vi "ACT_Loop_Single Test.vi"() -> ()   [LabVIEW 2023]
uses:
  Cluster_CMD_ACT_Data.ctl
  Shared Code/TypeDefs/ENUM_CMD_Mode Select.ctl
  Shared Code/TypeDefs/Cluster_CMD_Direction Data.ctl
  Shared Code/TypeDefs/Cluster_Module Velocity-Direction-Rotations.ctl
  Shared Code/TypeDefs/Level_Velocity plus-minus 1.ctl
  Shared Code/TypeDefs/Dial_Compase heading unit circle CCW positive.ctl
  Shared Code/TypeDefs/Cluster_X-Y.ctl
  <vilib>/Rock Robotics/WPI/ThirdParty/REV Robotics/REVLib/Typedef/Spark MAX Control Type.ctl
  Type Defs/ENUM_Steer Mode Select.ctl
  Shared Code/TypeDefs/Cluster_Swerve 4 Steer and Velocity.ctl
  Shared Code/TypeDefs/Cluster_Swerve Actual Settings.ctl
  Shared Code/TypeDefs/Cluster_Module Actual Settings.ctl
  Shared Code/TypeDefs/Dial_Actual Direction.ctl
  ENUM_ACT_State.ctl
  <vilib>/Rock Robotics/WPI/MotorControl/WPI_MotorControlDeviceRef.ctl
  <vilib>/Rock Robotics/WPI/MotorControl/WPI_MotorControlType.ctl
  <vilib>/Rock Robotics/SystemInterfaces/DIO/FPGA_DIOPWMChannel.ctl
  <vilib>/Rock Robotics/WPI/PWM/WPI_PWMDeadband.ctl
  <vilib>/Rock Robotics/SystemInterfaces/DIO/FPGA_DIOChannel.ctl
  Shared Code/TypeDefs/ENUM_Module Position.ctl
  Type Defs/Cluster_Avoid Zone.ctl
  Shared Code/TypeDefs/Cluster_Config_Swerve Drive Parameters.ctl
  Type Defs/Cluster_Length and Width.ctl
  Shared Code/TypeDefs/Cluster_Config_SwerveParam Steer.ctl
  Shared Code/TypeDefs/Cluster_Config_SwerveParam Drive.ctl
  <vilib>/Rock Robotics/WPI/ThirdParty/Phoenix-LabVIEW/CANCoder/Controls/CTRE_Phoenix_CANcoder_DeviceRef.ctl
  ENUM_ACT_Action.ctl
  RoboRIO Utilities/Global_STOP.vi
  Global_CMD_ACT_Data In.vi
  PigeonIMU/Global_SEN_Data Out.vi
  <vilib>/Rock Robotics/WPI/ThirdParty/Phoenix-LabVIEW/CANCoder/Get/CTRE_Phoenix_CANcoder_GetSensorData.vi
  Global_ACT_Data Out.vi
  SwerveDrive_ACT_ts.lvlib
  PigeonIMU/PigeonIMU_SEN_ts.lvlib
panel:
  in  "OVERIDE Tab":enum32{"Teleop-Auto", "Move", "Stop"}(tab)
  in  "SEND CMD(Momentry)":bool
  in  "Rotation Reduction 1-0":dbl=0.5
  in  "Orientation Robot(t) Field(f)":bool=TRUE
  in  "Direction":T1 {"Rotate(Yaw) CCW 1 CW -1" scale=1.0..-1.0; "Traverse"."Angle" scale format="%.3f"; "Traverse"."Velocity" scale=-1.0..1.0 scale format="%.1f"}
  in  "Max Translation Speed (ft/sec)":dbl
  out "Cancoder Values":dbl[](array[numeric]) format="%#.6f"
  out "Steer values":dbl[](array[numeric]) format="%.6g"
  out "unit circ Steer values":dbl[](array[numeric]) format="%.6g"
  out "unit circ Cancoder values":dbl[](array[numeric]) format="%#.6f"
  out "Yaw":T4 scale format="%.3f"
  out "Swerve SET Actual":T5 {"Back Right"."Encoder" format="%.2f"; "Back Right"."Direction" scale format="%.3f"; "Back Right"."Velocity" format="%.2f"; "Back Left"."Encoder" format="%.2f"; "Back Left"."Direction" scale format="%.3f"; "Back Left"."Velocity" format="%.2f"; "Front Left"."Encoder" format="%.2f"; "Front Left"."Direction" scale format="%.3f"; "Front Left"."Velocity" format="%.2f"; "Front Right"."Encoder" format="%.2f"; "Front Right"."Direction" scale format="%.3f"; "Front Right"."Velocity" format="%.2f"}
  out "calc time":dbl
  out "Swerve Set":T8 {"Back Right"."Angle" scale format="%.3f"; "Back Right"."Velocity" scale=-1.0..1.0 scale format="%.1f"; "Back Left"."Angle" scale format="%.3f"; "Back Left"."Velocity" scale=-1.0..1.0 scale format="%.1f"; "Front Left"."Angle" scale format="%.3f"; "Front Left"."Velocity" scale=-1.0..1.0 scale format="%.1f"; "Front Right"."Angle" scale format="%.3f"; "Front Right"."Velocity" scale=-1.0..1.0 scale format="%.1f"}
  out "Max Velocity(RPM)":dbl=200.0
  out "Steer Mode":T9
  out "Max Velocity FPS":dbl=2.0
  out "Drive Control Mode":T10
  out "Input CMD":T11 {"Auto Angle" scale format="%.3f"; "Direction"."Rotate(Yaw) CCW 1 CW -1" scale=1.0..-1.0; "Direction"."Traverse"."Angle" scale format="%.3f"; "Direction"."Traverse"."Velocity" scale=-1.0..1.0 scale format="%.1f"}
  out "Cycle Time (S)":dbl format="%.3g"
  # "TeleOp or Auto Control"
  # "STOP"
  # "\"Front\" of Robot"
  # "X"
  # "+CCW"
  # "Y"
  # "(0,0)"
  # "\"Front\" of Robot"
  # "Right Hand Rule"
  # "X"
  # "+CCW"
  # "Y"
  # "(0,0)"
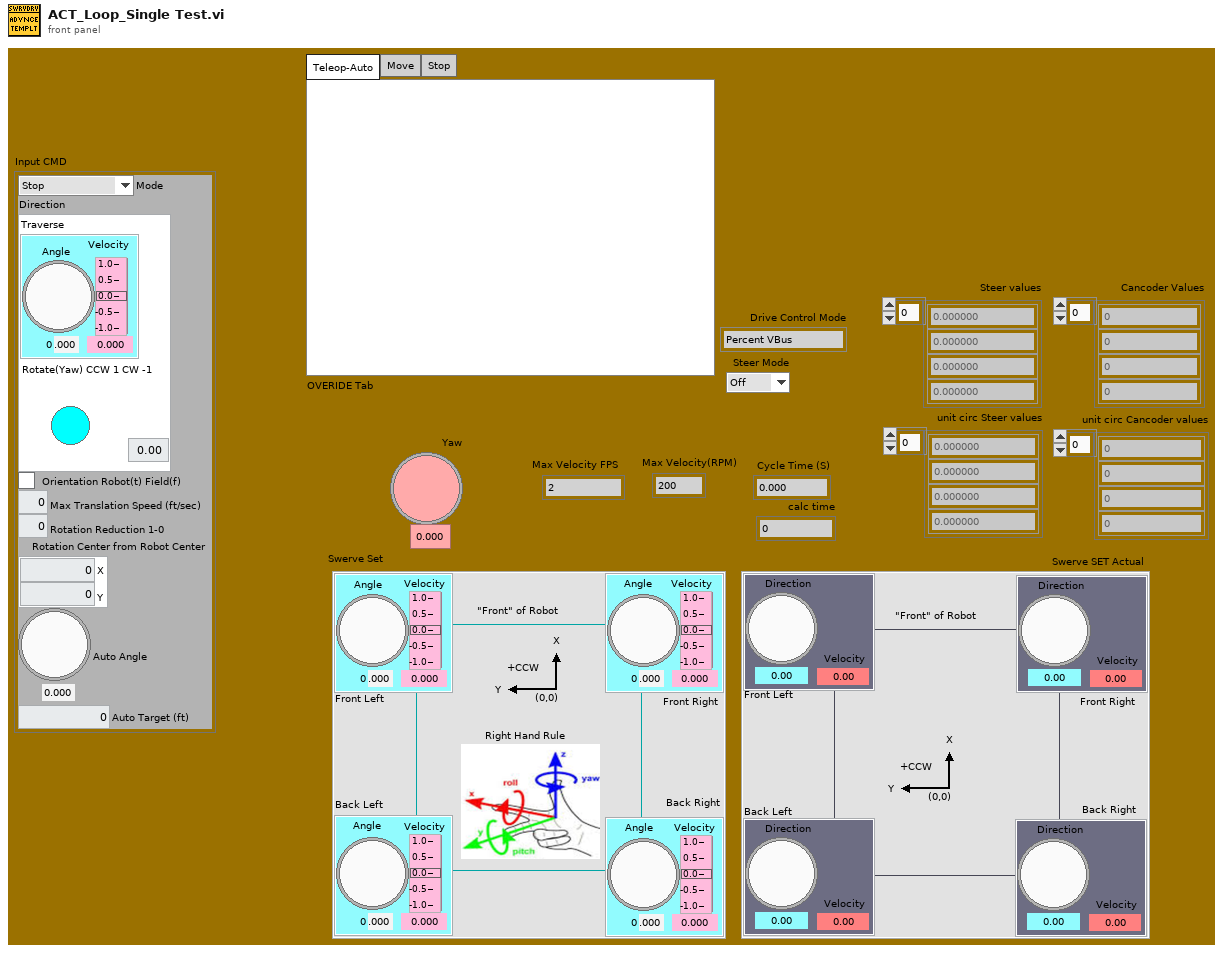
[diagram p1: front panel]
types:
  T1 = typedef "Cluster_CMD_Direction Data.ctl" = cluster{"Traverse":T2, "Rotate(Yaw) CCW 1 CW -1":dbl}
  T2 = typedef "Cluster_Module Velocity-Direction-Rotations.ctl" = cluster{"Velocity":T3, "Angle":T4, "Rotations Count":dbl}
  T3 = typedef "Level_Velocity plus-minus 1.ctl" = dbl
  T4 = typedef "Dial_Compase heading unit circle CCW positive.ctl" = dbl
  T5 = typedef "Cluster_Swerve Actual Settings.ctl" = cluster{"Front Right":T6, "Front Left":T6, "Back Left":T6, "Back Right":T6}
  T6 = typedef "Cluster_Module Actual Settings.ctl" = cluster{"Velocity":dbl, "Direction":T7, "Encoder":dbl}
  T7 = typedef "Dial_Actual Direction.ctl" = dbl
  T8 = typedef "Cluster_Swerve 4 Steer and Velocity.ctl" = cluster{"Front Right":T2, "Front Left":T2, "Back Left":T2, "Back Right":T2}
  T9 = typedef "ENUM_Steer Mode Select.ctl" = enum16{"Off", "Hold", "Steer"}
  T10 = typedef "Spark MAX Control Type.ctl" = enum16{"Percent VBus", "Voltage", "Velocity", "Position", "Smart Motion", "Current", "Smart Velocity"}
  T11 = typedef "SwerveDrive_ACT_ts.lvlib/Cluster_CMD_ACT_Data.ctl" = cluster{"Mode":T12, "Direction":T1, "Orientation Robot(t) Field(f)":bool, "Max Translation Speed (ft/sec)":dbl, "Rotation Reduction 1-0":dbl, "Rotation Center from Robot Center":T13, "Auto Angle":T4, "Auto Target (ft)":dbl}
  T12 = typedef "ENUM_CMD_Mode Select.ctl" = enum16{"Stop", "Move", "Turret Manual"}
  T13 = typedef "Cluster_X-Y.ctl" = cluster{"X":dbl, "Y":dbl}
  T14 = typedef "CTRE_Phoenix_CANcoder_DeviceRef.ctl" = cluster{"DeviceStatus":errorcluster, "Device Number":u8, "Handle":u64, "UsageFrame":u32, "Library Path":path}
  T15 = typedef "Cluster_Config_Swerve Drive Parameters.ctl" = cluster{"SwerveParam Ver":u64, "Frame":T16, "Steer":T17, "Drive":T18}
  T16 = typedef "Cluster_Length and Width.ctl" = cluster{"Length":dbl, "Width":dbl}
  T17 = typedef "Cluster_Config_SwerveParam Steer.ctl" = cluster{"CPR":dbl}
  T18 = typedef "Cluster_Config_SwerveParam Drive.ctl" = cluster{"CPR":dbl, "RevMotor/Wheel":dbl, "Wheel Diameter (in)":dbl}
  T19 = typedef "Cluster_Avoid Zone.ctl" = cluster{"pos 1":dbl, "pos 2":dbl}
  T20 = typedef "ENUM_Module Position.ctl" = enum16{"Left-Front", "Right-Front", "Left-Back", "Right-Back"}
  T21 = typedef "WPI_MotorControlDeviceRef.ctl" = cluster{"DeviceStatus":errorcluster, "Type":T22, "PWM":cluster{"PWM Channel":T23, "DeadBand":T24}, "CAN":cluster{"Device Number":u8, "SetOutput VI Ref":variant, "GetOutput VI Ref":variant, "Enable VI Ref":variant, "Disable VI Ref":variant, "Data":variant}, "Invert":bool, "DIO PWM":cluster{"PWM \"Enable\" Channel":T23, "DIOChannel":T25, "PWM Rate":dbl}}
  T22 = typedef "WPI_MotorControlType.ctl" = enum16{"PWM", "CAN", "DIO PWM"}
  T23 = typedef "FPGA_DIOPWMChannel.ctl" = enum8{"PWM 0", "PWM 1", "PWM 2", "PWM 3", "PWM 4", "PWM 5", "PWM 6", "PWM 7", "PWM 8", "PWM 9", "PWM MXP 0", "PWM MXP 1", "PWM MXP 2", "PWM MXP 3", "PWM MXP 4", "PWM MXP 5", "PWM MXP 6", "PWM MXP 7", "PWM MXP 8", "PWM MXP 9", "Invalid"}
  T24 = typedef "WPI_PWMDeadband.ctl" = cluster{"Name":string, "maxPositivePwm":i32, "minPositivePwm":i32, "centerPwm":i32, "maxNegativePwm":i32, "minNegativePwm":i32, "angularRange":u16}
  T25 = typedef "FPGA_DIOChannel.ctl" = enum8{"DIO 0", "DIO 1", "DIO 2", "DIO 3", "DIO 4", "DIO 5", "DIO 6", "DIO 7", "DIO 8", "DIO 9", "DIO MXP 0", "DIO MXP 1", "DIO MXP 2", "DIO MXP 3", "DIO MXP 4", "DIO MXP 5", "DIO MXP 6", "DIO MXP 7", "DIO MXP 8", "DIO MXP 9", "DIO MXP 10", "DIO MXP 11", "DIO MXP 12", "DIO MXP 13", "DIO MXP 14", "DIO MXP 15", "SPI Port CS1", "SPI Port CS2", "SPI Port CS3", "SPI Port MISO", "SPI Port MOSI", "Invalid"}
  T26 = typedef "SwerveDrive_ACT_ts.lvlib/ENUM_ACT_State.ctl" = enum16{"Startup", "Stopping", "Moving", "Shutdown"}
  T27 = typedef "SwerveDrive_ACT_ts.lvlib/ENUM_ACT_Action.ctl" = enum16{"No Action", "Reset Time", "Reset All", "2 Pos Set Direction", "2 Pos Set Speed", "Record Data", "Set Move from Values", "Reset Steer to Absolute"}
  T28 = cluster{"Motor List":T20[], "Drive Refs":T21[], "Steer Refs":T21[], "State":T26, "Previous State":T26, "Current Time":timestamp, "Previous Time":timestamp, "Start Time":timestamp, "Target Time (ms)":u32, "Cycle Time(S)":dbl, "ACT Input":T11, "Drive Control Mode":T10, "Drive PID Slot":i32, "Steer Position Values":dbl[], "Drive Velocity Values":dbl[], "Steer Position Times":dbl[], "Drive Velocity Times":dbl[], "Stream":bool, "Drive Output Times":dbl[], "Drive Output Values":dbl[], "Zero Start Steer Positions":dbl[], "Steer Mode":T9, "Max Velocity RPM":dbl, "Avoid Zone":T19, "Swerve Set":T8, "calc Start Time":dbl, "Compass Heading":T4, "Swerve Config ":T15, "Team Folder":path, "Steer Output Times":dbl[], "Can Coder Refs":T14[], "Can Coder Output postions":dbl[]}
  T29 = typedef "Cluster_Unity Yaw-Pitch-Roll.ctl" = cluster{"Yaw":T4, "Pitch":T4, "Roll":T4}
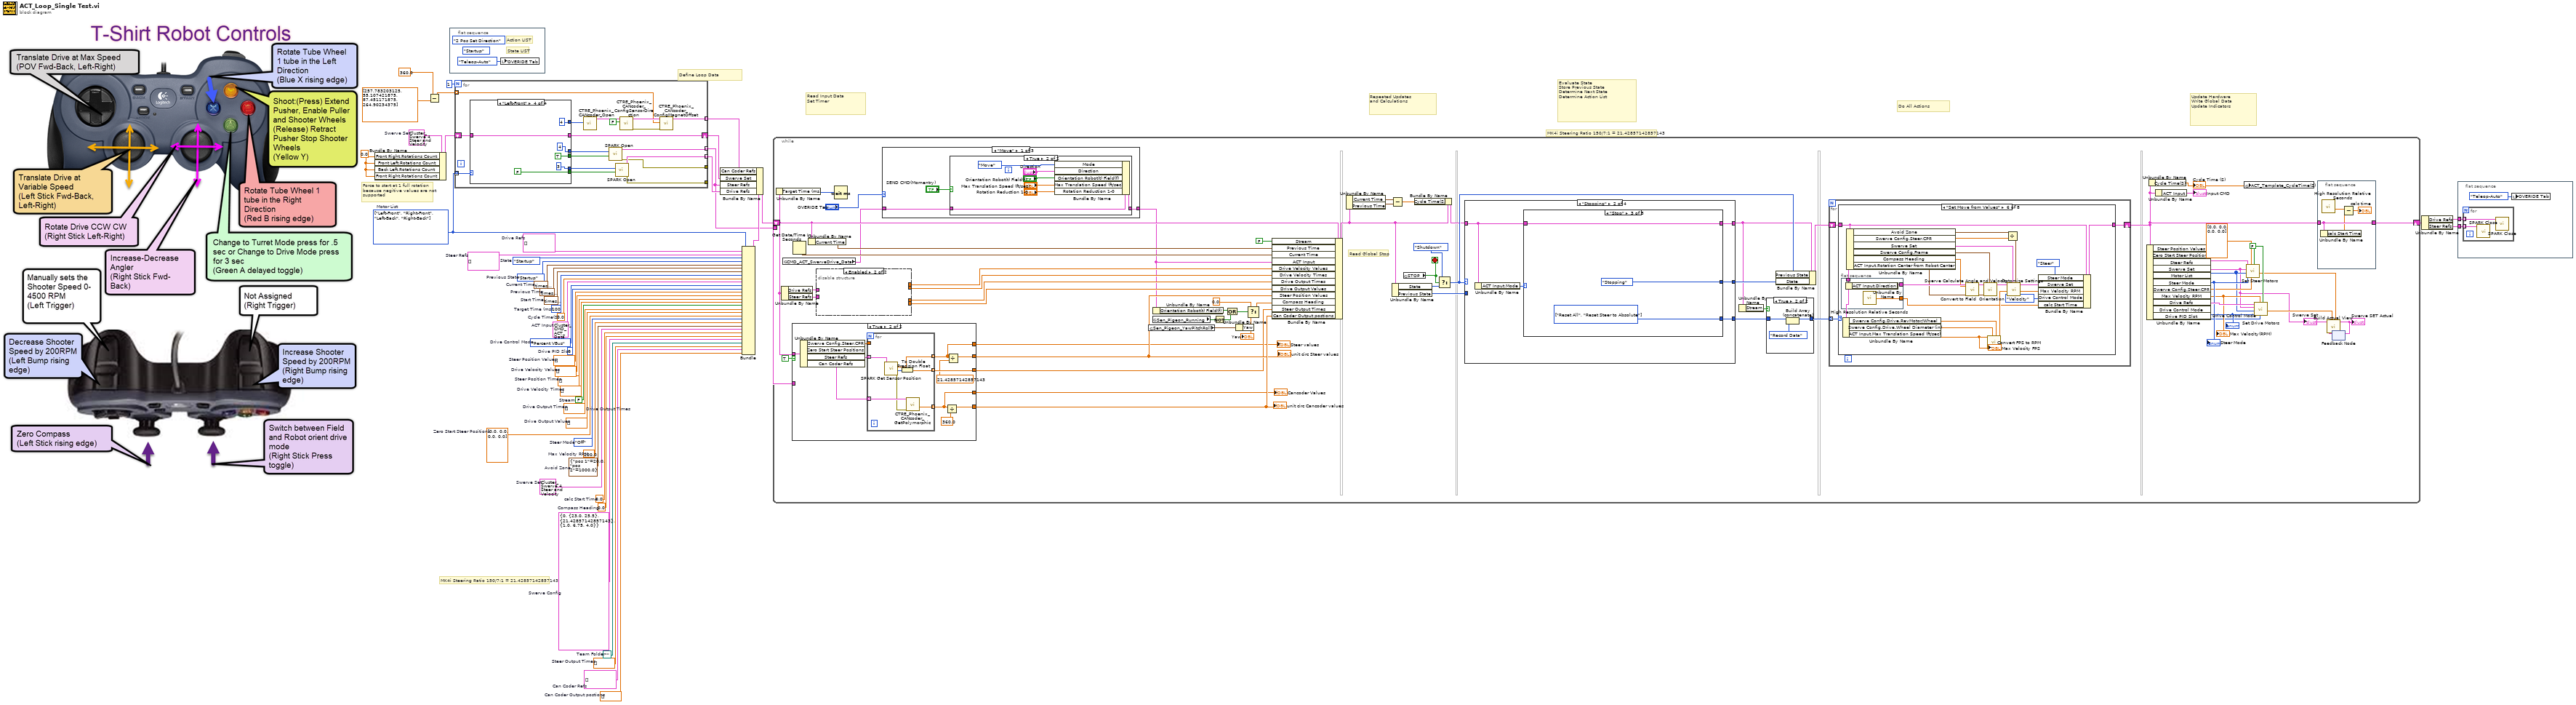
[diagram p0: block diagram]
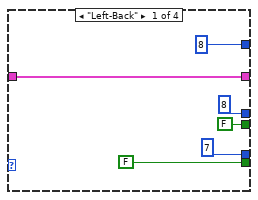
[diagram p2: hidden frame]
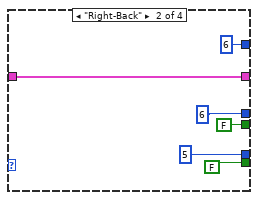
[diagram p3: hidden frame]
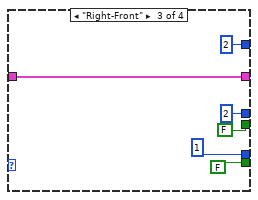
[diagram p4: hidden frame]
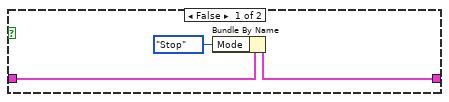
[diagram p5: hidden frame]
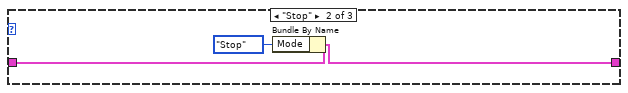
[diagram p6: hidden frame]
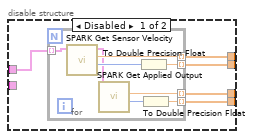
[diagram p8: hidden frame]
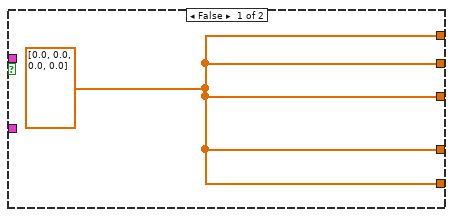
[diagram p9: hidden frame]
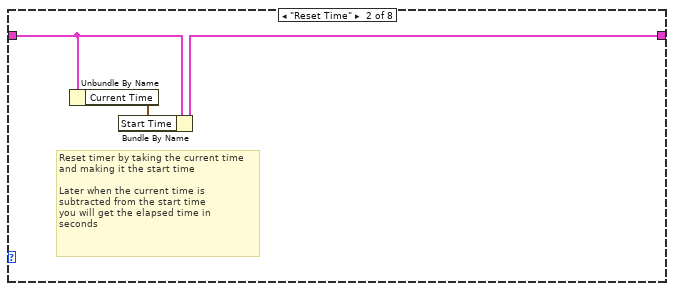
[diagram p12: hidden frame]
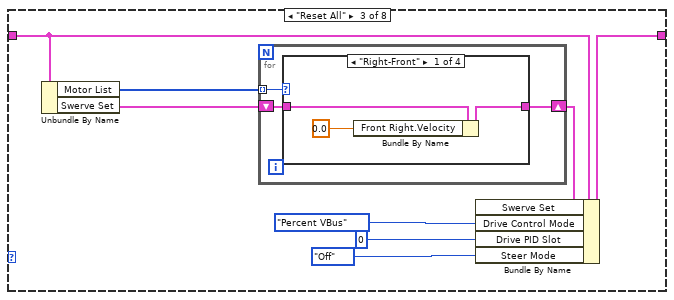
[diagram p13: hidden frame]
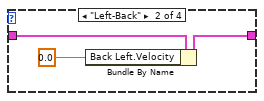
[diagram p14: hidden frame]
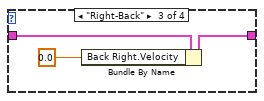
[diagram p15: hidden frame]
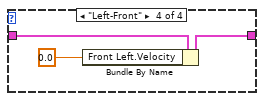
[diagram p16: hidden frame]
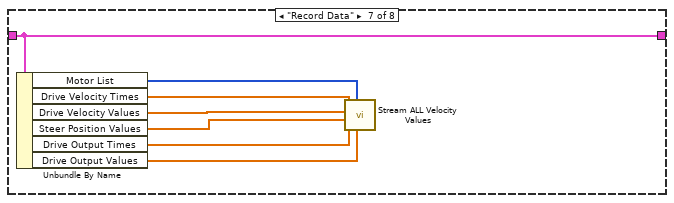
[diagram p19: hidden frame]
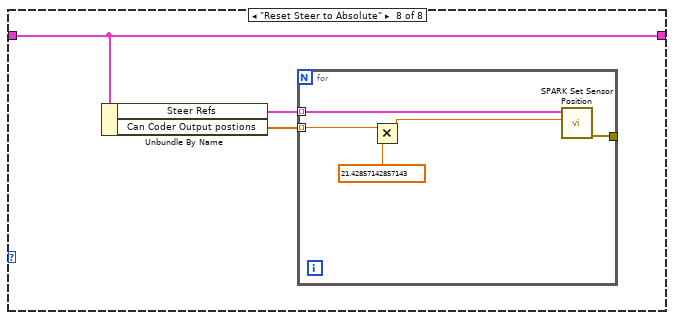
[diagram p20: hidden frame]
diagram:
  w2 = 0.0
  w9 = dbl[] []  # Can Coder Output postions
  w11 = T14[] []  # Can Coder Refs
  w12 = dbl[] []  # Steer Output Times
  (unwired) dbl[] []  # Drive Output Times
  w13 = path ""  # Team Folder
  w14 = T15 {"SwerveParam Ver"=0, "Frame"={"Length"=23.0, "Width"=25.5}, "Steer"={"CPR"=21.42857142857143}, "Drive"={"CPR"=1.0, "RevMotor/Wheel"=6.75, "Wheel Diameter (in)"=4.0}}  # Swerve Config
  w15 = T4 0.0  # Compass Heading
  w16 = 0.0  # calc Start Time
  w4 = T8 {"Front Right"={"Velocity"=0.0, "Angle"=0.0, "Rotations Count"=0.0}, "Front Left"={"Velocity"=0.0, "Angle"=0.0, "Rotations Count"=0.0}, "Back Left"={"Velocity"=0.0, "Angle"=0.0, "Rotations Count"=0.0}, "Back Right"={"Velocity"=0.0, "Angle"=0.0, "Rotations Count"=0.0}}  # Swerve Set
  w18 = T8 {"Front Right"={"Velocity"=0.0, "Angle"=0.0, "Rotations Count"=0.0}, "Front Left"={"Velocity"=0.0, "Angle"=0.0, "Rotations Count"=0.0}, "Back Left"={"Velocity"=0.0, "Angle"=0.0, "Rotations Count"=0.0}, "Back Right"={"Velocity"=0.0, "Angle"=0.0, "Rotations Count"=0.0}}  # Swerve Set
  w19 = T19 {"pos 1"=20.0, "pos 2"=1000.0}  # Avoid Zone
  w20 = T20[] [enum."Left-Front", enum."Right-Front", enum."Left-Back", enum."Right-Back"] items=["Left-Front", "Right-Front", "Left-Back", "Right-Back"]  # Motor List
  w21 = 200.0  # Max Velocity RPM
  w22 = ENUM_Steer_Mode_Select."Off"  # Steer Mode
  w23 = dbl[] [0.0, 0.0, 0.0, 0.0]  # Zero Start Steer Positions
  w24 = dbl[] []  # Drive Output Values
  w25 = dbl[] []  # Drive Output Times
  w26 = FALSE  # Stream
  w27 = dbl[] []  # Drive Velocity Times
  w28 = dbl[] []  # Steer Position Times
  w29 = dbl[] []  # Drive Velocity Values
  w30 = dbl[] []  # Steer Position Values
  w33 = 0  # Drive PID Slot
  w34 = Spark_MAX_Control_Type."Percent VBus"  # Drive Control Mode
  w38 = T21[] []  # Drive Refs
  w39 = T21[] []  # Steer Refs
  w41 = 0.0  # Cycle Time(S)
  w42 = ENUM_ACT_State."Startup"  # Previous State
  w43 = timestamp(0 s since 1904-01-01)  # Previous Time
  w44 = u32 100  # Target Time (ms)
  w45 = T11 {"Mode"=enum."Stop", "Direction"={"Traverse"={"Velocity"=0.0, "Angle"=0.0, "Rotations Count"=0.0}, "Rotate(Yaw) CCW 1 CW -1"=0.0}, "Orientation Robot(t) Field(f)"=FALSE, "Max Translation Speed (ft/sec)"=0.0, "Rotation Reduction 1-0"=0.0, "Rotation Center from Robot Center"={"X"=0.0, "Y"=0.0}, "Auto Angle"=0.0, "Auto Target (ft)"=0.0}  # ACT Input
  w46 = timestamp(0 s since 1904-01-01)  # Start Time
  w47 = timestamp(0 s since 1904-01-01)  # Current Time
  w48 = ENUM_ACT_State."Startup"  # State
  # "Force to start at 1 full rotation\nbecause negitive values are not\nsupported"
  # "MK4i Steering Ratio 150/7:1 = 21.42857142857143"
  # "MK4i Steering Ratio 150/7:1 = 21.42857142857143"
  # "Define Loop Data"
  # "Repeated Updates\nand Calculations"
  # "Read Input Data\nSet Timer"
  # "Evaluate State\nStore Previous State\nDetermine Next State\nDetermine Action List"
  # "Do All Actions"
  # "Update Hardware\nWrite Global Data\nUpdate Indicators"
  n1 = Bundle By Name(cluster=w4, "Front Right.Rotations Count"=w2, "Front Left.Rotations Count"=w2, "Back Left.Rotations Count"=w2, "Front Right.Rotations Count"=w2) -> (w3:T8)
  n2 = Subtract(x=360.0, y=dbl[] [257.783203125, 55.107421875, 87.451171875, 264.90234375] ("Cancoder Values")) -> (x-y=w5:dbl[])
  n3 = flat-sequence {
    frame #0 {
      (unwired) ENUM_ACT_State."Startup" ("State")
      (unwired) ENUM_ACT_Action."2 Pos Set Direction" ("Action")
      # "State LIST"
      # "Action LIST"
      n4 = local write "OVERIDE Tab"(enum32{"Teleop-Auto", "Move", "Stop"}."Teleop-Auto" ("OVERIDE Tab")) -> ()
    }
  }
  n5 = for {
    N: 1 ("Numeric") -> [_]
    tunnel: w20 -> [w67] mode=indexing
    tunnel: [w61] -> w8 mode=indexing
    tunnel: [w64] -> w35 mode=indexing
    shift-right: [w65] -> w17
    shift-left: w3 -> [w66]
    tunnel: [w63] -> _
    tunnel: [w52] -> w10 mode=indexing
    tunnel: [w56] -> _
    tunnel: w5 -> [w50] mode=indexing
    n6 = case shown="\"Left-Front\"" w67 {
      tunnel: [FALSE ("Invert") FALSE ("Invert") FALSE ("Invert") FALSE ("Invert")] -> w62
      tunnel: [u8 7 ("unsigned 8bit integer") u8 5 ("unsigned 8bit integer") u8 1 ("unsigned 8bit integer") u8 3 ("unsigned 8bit integer")] -> w60
      tunnel: w66 -> [w68 w74 w80 w86]
      tunnel: [w68 w74 w80 w86] -> w65
      tunnel: [u8 8 ("Device Number") u8 6 ("Device Number") u8 2 ("Device Number") u8 4 ("Device Number")] -> w59
      tunnel: [FALSE ("Invert") FALSE ("Invert") FALSE ("Invert") TRUE ("Invert")] -> w58
      tunnel: [u8 8 ("Device Number") u8 6 ("Device Number") u8 2 ("Device Number") u8 4 ("Device Number")] -> w57
      frame "Left-Back" {
      }
      frame "Right-Back" {
      }
      frame "Right-Front" {
      }
      frame "Left-Front" {
      }
    }
    n7 = call <vilib>:"CTRE_Phoenix_CANcoder_Open.vi"("Device Number"=w57) -> ("CTRE_CANcoder_DeviceRef"=w55:T14)  [unwired: 9 in, 1 out]
    n8 = call <vilib>:"SPARK Open.vi"("Invert"=w58, "Device Number"=w59) -> ("error out"=w56:errorcluster, "MotorControlDeviceRef"=w61:T21)  [unwired: 8 in]
    n9 = call <vilib>:"SPARK Open.vi"("Invert"=w62, "Device Number"=w60) -> ("error out"=w63:errorcluster, "MotorControlDeviceRef"=w64:T21)  [unwired: 8 in]
    n10 = call <vilib>:"CTRE_Phoenix_CANcoder_ConfigSensorDirection.vi"("Sensor Direction"=FALSE, "CTRE_CANcoder_DeviceRef"=w55) -> ("error out"=w51:errorcluster, "CTRE_CANcoder_DeviceRef"=w53:T14)  [unwired: 8 in]
    n11 = call <vilib>:"CTRE_Phoenix_CANcoder_ConfigMagnetOffset.vi"("error in"=w51, "Magnet Offset (Degrees)"=w50, "CTRE_CANcoder_DeviceRef"=w53) -> ("CTRE_CANcoder_DeviceRef"=w52:T14)  [unwired: 7 in, 1 out]
  }
  n12 = Bundle("Motor List"=w20, "Drive Refs"=w38, "Steer Refs"=w39, "State"=w48, "Previous State"=w42, "Current Time"=w47, "Previous Time"=w43, "Start Time"=w46, "Target Time (ms)"=w44, "Cycle Time(S)"=w41, "ACT Input"=w45, "Drive Control Mode"=w34, "Drive PID Slot"=w33, "Steer Position Values"=w30, "Drive Velocity Values"=w29, "Steer Position Times"=w28, "Drive Velocity Times"=w27, "Stream"=w26, "Drive Output Times"=w25, "Drive Output Values"=w24, "Zero Start Steer Positions"=w23, "Steer Mode"=w22, "Max Velocity RPM"=w21, "Avoid Zone"=w19, "Swerve Set"=w18, "calc Start Time"=w16, "Compass Heading"=w15, "Swerve Config"=w14, "Team Folder"=w13, "Steer Output Times"=w12, "Can Coder Refs"=w11, "Can Coder Output postions"=w9) -> (w37:T28)  [unwired: 1 in]
  n13 = Bundle By Name(cluster=w37, "Can Coder Refs"=w10, "Swerve Set"=w17, "Steer Refs"=w8, "Drive Refs"=w35) -> (w36:T28)
  n14 = while {
    shift-right: [w99] -> w40
    shift-left: w36 -> [w127]
    tunnel: w8 -> [w100]
    stop <- w152 stop-if-true
    w116 = FALSE
    # "Read Global Stop"
    n15 = Unbundle By Name(w127) -> ("Target Time (ms)"=w149:u32)
    n16 = Unbundle By Name(w127) -> ("Drive Refs"=w126:T21[], "Steer Refs"=w98:T21[])
    n17 = global read "Global_CMD_ACT_Data In.vi" "CMD_ACT_SwerveDrive_Data"() -> (w95:T11)
    n18 = case shown="True" TRUE {
      tunnel: [w190 w194] -> w102
      tunnel: w127 -> [_ w201]
      tunnel: [w190 w195] -> w101
      tunnel: [w190 w197] -> w103
      tunnel: w100 -> [_ _]
      tunnel: [w190 w192] -> w97
      tunnel: [w190 w191] -> w96
      frame False {
        w190 = dbl[] [0.0, 0.0, 0.0, 0.0]
      }
      frame True {
        n19 = Unbundle By Name(w201) -> ("Swerve Config.Steer.CPR"=w200:dbl, "Steer Refs"=w198:T21[], "Can Coder Refs"=w199:T14[])  [unwired: 1 out]
        n20 = for {
          tunnel: [w203] -> w192 mode=indexing
          tunnel: w200 -> [_]
          tunnel: [w207] -> w195 mode=indexing
          tunnel: w199 -> [w206] mode=indexing
          tunnel: [w205] -> w191 mode=indexing
          tunnel: w198 -> [w204] mode=indexing
          n21 = call <vilib>:"SPARK Get Sensor Position.vi"("MotorControlDevRef in"=w204) -> ("error out"=w202:errorcluster, "Timestamp"=w208:u32, "Sensor Position"=w203:dbl)  [unwired: 7 in, 1 out]
          n22 = To Double Precision Float(number=w208) -> (double precision float=w207:dbl)
          n23 = call-poly <vilib>:"CTRE_Phoenix_CANcoder_GetPolymorphic.vi"("CTRE_CANcoder_DeviceRef"=w206, "error in"=w202) -> ("Absolute Position"=w205:dbl)  [unwired: 9 in, 4 out]
        }
        n24 = Divide(x=w191, y=360.0 ("Absolute Position")) -> (x/y=w197:dbl[])
        n25 = Divide(x=w192, y=21.42857142857143 ("Absolute Position")) -> (x/y=w194:dbl[])
      }
    }
    "unit circ Cancoder values" <- w103
    "unit circ Steer values" <- w102
    "Steer values" <- w97
    "Cancoder Values" <- w96
    n26 = Get Date/Time In Seconds() -> (seconds since 1Jan1904=w155:timestamp)
    n27 = Unbundle By Name(w127) -> ("Current Time"=w148:timestamp)
    n28 = disable-structure shown="Enabled" {
      disable-tunnel: [w177 _] -> w136
      disable-tunnel: [w176 _] -> w135
      disable-tunnel: [w175 _] -> w133
      disable-tunnel: [w174 _] -> w132
      disable-tunnel: w126 -> [w173 _]
      disable-tunnel: w98 -> [_ _]
      frame Disabled {
        n29 = for {
          tunnel: w173 -> [w183] mode=indexing
          tunnel: [w182] -> w177 mode=indexing
          tunnel: [w185] -> w176 mode=indexing
          tunnel: [w179] -> w175 mode=indexing
          tunnel: [w184] -> w174 mode=indexing
          n30 = call <vilib>:"SPARK Get Sensor Velocity.vi"("MotorControlDevRef in"=w183) -> ("Timestamp"=w181:u32, "Sensor Velocity"=w182:dbl, "MotorControlDevRef out"=w180:T21)  [unwired: 7 in, 1 out]
          n31 = call <vilib>:"SPARK Get Applied Output.vi"("MotorControlDevRef in"=w180) -> ("Timestamp"=w178:u32, "Applied Output"=w179:dbl)  [unwired: 7 in, 2 out]
          n32 = To Double Precision Float(number=w181) -> (double precision float=w185:dbl)
          n33 = To Double Precision Float(number=w178) -> (double precision float=w184:dbl)
        }
      }
      frame Enabled {
      }
    }
    n34 = Wait (ms)(milliseconds to wait=w149) -> ()  [unwired: 1 out]
    n35 = case shown="\"Move\"" "OVERIDE Tab" {
      tunnel: w95 -> [w157 w171 w172]
      tunnel: [w156 w170 w172] -> w94
      frame "Move" {
        n36 = case shown="True" "SEND CMD(Momentry)" {
          tunnel: w157 -> [w161 w168]
          tunnel: [w160 w167] -> w156
          frame False {
            n37 = Bundle By Name(cluster=w161, "Mode"=ENUM_CMD_Mode_Select."Stop") -> (w160:T11)
          }
          frame True {
            n38 = Bundle By Name(cluster=w168, "Mode"=ENUM_CMD_Mode_Select."Move", "Direction"="Direction", "Orientation Robot(t) Field(f)"="Orientation Robot(t) Field(f)", "Max Translation Speed (ft/sec)"="Max Translation Speed (ft/sec)", "Rotation Reduction 1-0"="Rotation Reduction 1-0") -> (w167:T11)
          }
        }
      }
      frame "Stop" {
        n39 = Bundle By Name(cluster=w171, "Mode"=ENUM_CMD_Mode_Select."Stop") -> (w170:T11)
      }
      frame "Teleop-Auto" {
      }
    }
    n40 = global read "Global_SEN_Data Out.vi" "Sen_Pigeon_YawPitchRoll"() -> (w110:T29)
    n41 = global read "Global_SEN_Data Out.vi" "Sen_Pigeon_Running"() -> (w106:bool)
    n42 = Unbundle By Name(w94) -> ("Orientation Robot(t) Field(f)"=w112:bool)
    n43 = Not(x=w106) -> (.not. x?=w105:bool)
    n44 = Or(x=w112, y=w105) -> (x .or. y?=w107:bool)
    n45 = Unbundle By Name(w110) -> ("Yaw"=w109:T4)
    "Yaw" <- w109
    n46 = Select(t=T4 0.0, s=w107, f=w109) -> (s? t:f=w111:T4)
    n47 = Bundle By Name(cluster=w127, "Stream"=FALSE, "Previous Time"=w148, "Current Time"=w155, "ACT Input"=w94, "Drive Velocity Values"=w136, "Drive Velocity Times"=w135, "Drive Output Times"=w133, "Drive Output Values"=w132, "Steer Position Values"=w102, "Compass Heading"=w111, "Steer Output Times"=w101, "Can Coder Output postions"=w103) -> (w143:T28)
    n48 = Unbundle By Name(w143) -> ("Current Time"=w144:timestamp, "Previous Time"=w145:timestamp)
    n49 = Subtract(x=w144, y=w145) -> (x-y=w141:dbl)
    n50 = Unbundle By Name(w143) -> ("State"=w150:T26, "Previous State"=w147:T26)
    n51 = global read "Global_STOP.vi" "STOP"() -> (w152:bool)
    n52 = Bundle By Name(cluster=w143, "Cycle Time(S)"=w141) -> (w142:T28)
    n53 = Select(t=ENUM_ACT_State."Shutdown" ("State"), s=w152, f=w150) -> (s? t:f=w146:T26)
    n54 = case shown="\"Stopping\"" w146 {
      tunnel: w142 -> [w283 w290 w302 w318]
      tunnel: [w285 w291 w303 w318] -> w131
      tunnel: [ENUM_ACT_State."Moving" ("State") w292 w304 ENUM_ACT_State."Shutdown" ("State")] -> w153
      tunnel: [w287 w288 w300 w316] -> w129
      tunnel: w147 -> [_ _ _ _]
      frame "Startup" {
        w287 = T27[] [enum."Reset Steer to Absolute", enum."Reset Time", enum."Reset All", enum."Reset Steer to Absolute"] items=["No Action", "Reset Time", "Reset All", "2 Pos Set Direction", "2 Pos Set Speed", "Record Data", "Set Move from Values", "Reset Steer to Absolute"] ("Actions")
        n55 = Bundle By Name(cluster=w283, "Zero Start Steer Positions"=dbl[] []) -> (w285:T28)
      }
      frame "Stopping" {
        n56 = Unbundle By Name(w290) -> ("ACT Input.Mode"=w289:T12)
        n57 = case shown="\"Stop\"" w289 {
          tunnel: [ENUM_ACT_State."Moving" ("State") ENUM_ACT_State."Moving" ("State") ENUM_ACT_State."Stopping" ("State")] -> w292
          tunnel: [w293 w295 w297] -> w291
          tunnel: w290 -> [w293 w295 w297]
          tunnel: [_ _ w298] -> w288
          frame "Move" {
          }
          frame "Turret Manual" {
          }
          frame "Stop" {
            w298 = T27[] [enum."Reset All", enum."Reset Steer to Absolute"] items=["No Action", "Reset Time", "Reset All", "2 Pos Set Direction", "2 Pos Set Speed", "Record Data", "Set Move from Values", "Reset Steer to Absolute"] ("Actions")
          }
        }
      }
      frame "Moving" {
        n58 = Unbundle By Name(w302) -> ("ACT Input.Mode"=w301:T12)
        n59 = case shown="\"Turret Manual\"" w301 {
          tunnel: [ENUM_ACT_State."Moving" ("State") ENUM_ACT_State."Moving" ("State") ENUM_ACT_State."Stopping" ("State")] -> w304
          tunnel: [w306 w309 w314] -> w303
          tunnel: w302 -> [w306 w308 w314]
          tunnel: [w305 w311 w313] -> w300
          frame "Move" {
            w305 = T27[] [enum."Set Move from Values"] items=["No Action", "Reset Time", "Reset All", "2 Pos Set Direction", "2 Pos Set Speed", "Record Data", "Set Move from Values", "Reset Steer to Absolute"] ("Actions")
          }
          frame "Turret Manual" {
            w311 = T27[] [enum."Set Move from Values"] items=["No Action", "Reset Time", "Reset All", "2 Pos Set Direction", "2 Pos Set Speed", "Record Data", "Set Move from Values", "Reset Steer to Absolute"] ("Actions")
            n60 = Bundle By Name(cluster=w308, "ACT Input.Direction.Traverse.Velocity"=T3 0.0) -> (w309:T28)
          }
          frame "Stop" {
            w313 = T27[] [enum."Reset All"] items=["No Action", "Reset Time", "Reset All", "2 Pos Set Direction", "2 Pos Set Speed", "Record Data", "Set Move from Values", "Reset Steer to Absolute"] ("Actions")
          }
        }
      }
      frame "Shutdown" {
        w316 = T27[] [enum."Reset All"] items=["No Action", "Reset Time", "Reset All", "2 Pos Set Direction", "2 Pos Set Speed", "Record Data", "Set Move from Values", "Reset Steer to Absolute"] ("Actions")
      }
    }
    n61 = Unbundle By Name(w131) -> ("Stream"=w130:bool)
    n62 = case shown="True" w130 {
      tunnel: w129 -> [w209 w212]
      tunnel: [w209 w211] -> w128
      frame False {
      }
      frame True {
        n63 = Build Array (concatenate)(w212, ENUM_ACT_Action."Record Data" ("Action")) -> (w211:T27[])
      }
    }
    n64 = Bundle By Name(cluster=w131, "Previous State"=w146, "State"=w153) -> (w154:T28)
    n65 = for {
      tunnel: w128 -> [w215] mode=indexing
      shift-right: [w214] -> w118
      shift-left: w154 -> [w213]
      n66 = case shown="\"Set Move from Values\"" w215 {
        tunnel: w213 -> [w216 w219 w224 w243 w244 w260 w274 w277]
        tunnel: [w216 w218 w227 w243 w244 w264 w274 w277] -> w214
        frame "No Action" {
        }
        frame "Reset Time" {
          # "Reset timer by taking the current time\nand making it the start time\n\nLater when the current time is \nsubtracted from the start time\nyou will get the elapsed time in \nseconds"
          n67 = Unbundle By Name(w219) -> ("Current Time"=w217:timestamp)
          n68 = Bundle By Name(cluster=w219, "Start Time"=w217) -> (w218:T28)
        }
        frame "Reset All" {
          n69 = Unbundle By Name(w224) -> ("Motor List"=w222:T20[], "Swerve Set"=w221:T8)
          n70 = for {
            tunnel: w222 -> [w230] mode=indexing
            shift-right: [w228] -> w220
            shift-left: w221 -> [w229]
            n71 = case shown="\"Right-Front\"" w230 {
              tunnel: w229 -> [w233 w236 w239 w242]
              tunnel: [w232 w235 w238 w241] -> w228
              frame "Right-Front" {
                n72 = Bundle By Name(cluster=w233, "Front Right.Velocity"=T3 0.0 ("Front Right.Velocity (0-1)")) -> (w232:T8)
              }
              frame "Left-Back" {
                n73 = Bundle By Name(cluster=w236, "Back Left.Velocity"=T3 0.0 ("Front Right.Velocity (0-1)")) -> (w235:T8)
              }
              frame "Right-Back" {
                n74 = Bundle By Name(cluster=w239, "Back Right.Velocity"=T3 0.0 ("Front Right.Velocity (0-1)")) -> (w238:T8)
              }
              frame "Left-Front" {
                n75 = Bundle By Name(cluster=w242, "Front Left.Velocity"=T3 0.0 ("Front Right.Velocity (0-1)")) -> (w241:T8)
              }
            }
          }
          n76 = Bundle By Name(cluster=w224, "Swerve Set"=w220, "Drive Control Mode"=Spark_MAX_Control_Type."Percent VBus", "Drive PID Slot"=0, "Steer Mode"=ENUM_Steer_Mode_Select."Off") -> (w227:T28)
        }
        frame "2 Pos Set Direction" {
        }
        frame "2 Pos Set Speed" {
        }
        frame "Set Move from Values" {
          n77 = flat-sequence {
            tunnel: w260 -> [w267]
            tunnel: [w266] -> w248
            tunnel: [w265] -> w250
            frame #0 {
              n78 = Unbundle By Name(w267) -> ("ACT Input.Direction"=w266:T1)
              n79 = call <vilib>:"High Resolution Relative Seconds.vi"() -> ("relative seconds"=w265:dbl)
            }
          }
          n80 = Unbundle By Name(w260) -> ("Swerve Config.Drive.RevMotor/Wheel"=w258:dbl, "Swerve Config.Drive.Wheel Diameter (in)"=w259:dbl, "ACT Input.Max Translation Speed (ft/sec)"=w246:dbl)
          "Max Velocity FPS" <- w246
          n81 = Unbundle By Name(w260) -> ("Avoid Zone"=w256:T19, "Swerve Config.Steer.CPR"=w257:dbl, "Swerve Set"=w253:T8, "Swerve Config.Frame"=w251:T16, "Compass Heading"=w247:T4, "ACT Input.Rotation Center from Robot Center"=w245:T13)
          n82 = call "Convert to Field  Orientation.vi"("Compass Heading"=w247, "Direction in"=w248) -> ("Corrected Direction out"=w249:T1)  [unwired: 9 in]
          n83 = call "Swerve Calculate Angle and Velocity.vi"("Frame"=w251, "Rotation Center From Robot Center"=w245, "Comand Data"=w249) -> ("Swerve Request Out"=w255:T8)  [unwired: 8 in]
          n84 = call "Convert FPS to RPM.vi"("RevMotor/RevWheel"=w258, "Wheel Diameter (in)"=w259, "Translation Speed (ft/s)"=w246) -> ("Motor Speed (RPM) Out"=w261:dbl)  [unwired: 8 in]
          n85 = Divide(x=w256, y=w257) -> (x/y=w254:T19)
          n86 = call "Optomize Settings.vi"("Aviod Zone"=w254, "Previous Swerve Setting"=w253, "Swerve Request"=w255) -> ("Swerve Setting Out"=w252:T8)  [unwired: 8 in]
          n87 = Bundle By Name(cluster=w260, "Steer Mode"=ENUM_Steer_Mode_Select."Steer", "Swerve Set"=w252, "Max Velocity RPM"=w261, "Drive Control Mode"=Spark_MAX_Control_Type."Velocity", "calc Start Time"=w250) -> (w264:T28)
        }
        frame "Record Data" {
          n88 = Unbundle By Name(w274) -> ("Motor List"=w273:T20[], "Drive Velocity Times"=w272:dbl[], "Drive Velocity Values"=w271:dbl[], "Steer Position Values"=w270:dbl[], "Drive Output Times"=w269:dbl[], "Drive Output Values"=w268:dbl[])
          n89 = call "Stream ALL Velocity Values.vi"("Output Values"=w268, "Motor List"=w273, "Output Times"=w269, "Drive Target Values"=w270, "Drive Velocity Values"=w271, "Drive Times"=w272) -> ()  [unwired: 6 in]
        }
        frame "Reset Steer to Absolute" {
          n90 = Unbundle By Name(w277) -> ("Steer Refs"=w276:T21[], "Can Coder Output postions"=w275:dbl[])
          n91 = for {
            tunnel: w276 -> [w282] mode=indexing
            tunnel: w275 -> [w280] mode=indexing
            tunnel: [w281] -> _
            n92 = Multiply(x=w280, y=21.42857142857143 ("Absolute Position")) -> (x*y=w278:dbl)
            n93 = call <vilib>:"SPARK Set Sensor Position.vi"("Position"=w278, "MotorControlDeviceRef"=w282) -> ("error out"=w281:errorcluster)  [unwired: 8 in, 1 out]
          }
        }
      }
    }
    n94 = Unbundle By Name(w118) -> ("Steer Refs"=w138:T21[], "Swerve Set"=w104:T8, "Motor List"=w120:T20[], "Steer Mode"=w124:T9, "Swerve Config.Steer.CPR"=w121:dbl, "Max Velocity RPM"=w122:dbl, "Drive Refs"=w137:T21[], "Drive Control Mode"=w123:T10, "Drive PID Slot"=w119:i32)  [unwired: 2 out]
    "Drive Control Mode" <- w123
    "Steer Mode" <- w124
    "Max Velocity(RPM)" <- w122
    "Swerve Set" <- w104
    n95 = Unbundle By Name(w118) -> ("Cycle Time(S)"=w139:dbl)
    "Cycle Time (S)" <- w139
    n96 = Unbundle By Name(w118) -> ("ACT Input"=→"Input CMD":T11)
    n97 = global write "Global_ACT_Data Out.vi" "ACT_Template_CycleTime(S)"(w139) -> ()
    n98 = call "Set Steer Motors.vi"("Disable"=w116, "PPR"=w121, "Offset Encoder Positions"=dbl[] [0.0, 0.0, 0.0, 0.0], "Steer Control Mode"=w124, "Motor List"=w120, "Swerve Data"=w104, "Steer Refs"=w138) -> ("Encoder Counts Out"=w114:dbl[])  [unwired: 3 in, 1 out]
    n99 = call "Set Drive Motors.vi"("Disable"=w116, "Drive PID Slot"=w119, "Max Velocity(RPM)"=w122, "Drive Control Mode"=w123, "Motor List"=w120, "Swerve Data"=w104, "Drive Refs"=w137) -> ("Speeds"=w113:dbl[])  [unwired: 3 in, 1 out]
    n100 = flat-sequence {
      tunnel: w118 -> [w189]
      tunnel: [w189] -> w99
      frame #0 {
        n101 = Unbundle By Name(w189) -> ("calc Start Time"=w187:dbl)
        n102 = call <vilib>:"High Resolution Relative Seconds.vi"() -> ("relative seconds"=w188:dbl)
        n103 = Subtract(x=w188, y=w187) -> (x-y=→"calc time":dbl)
      }
    }
    n104 = feedback #1() -> (w115:T5)  [unwired: 1 in]
    n105 = call "Build Actual View.vi"("Encoder Counts Out"=w114, "Speeds"=w113, "Previous Actual"=w115, "Swerve Set"=w104) -> ("Swerve Data out"=w117:T5)  [unwired: 7 in]
    "Swerve SET Actual" <- w117
    n106 = feedback-in #1(w117) -> ()
  }
  n107 = Unbundle By Name(w40) -> ("Drive Refs"=w31:T21[], "Steer Refs"=w32:T21[])
  n108 = flat-sequence {
    tunnel: w32 -> [w321]
    tunnel: w31 -> [w320]
    frame #0 {
      n109 = for {
        tunnel: w321 -> [w323] mode=indexing
        tunnel: w320 -> [w322] mode=indexing
        n110 = call <vilib>:"SPARK Close.vi"("MotorControlDeviceRef"=w323) -> ()  [unwired: 10 in, 1 out]
        n111 = call <vilib>:"SPARK Close.vi"("MotorControlDeviceRef"=w322) -> ()  [unwired: 10 in, 1 out]
      }
      n112 = local write "OVERIDE Tab"(enum32{"Teleop-Auto", "Move", "Stop"}."Teleop-Auto" ("OVERIDE Tab")) -> ()
    }
  }
